vi "Build Type String.vi"(11 "App Build in":refnum<class "App Build.lvclass">) -> (2 "Build Type":string)   [LabVIEW 2020, in "Builder Tools.lvlib" / "App Build.lvclass"]
uses:
  App Build.lvclass
  App Build.lvclass/App Build.ctl
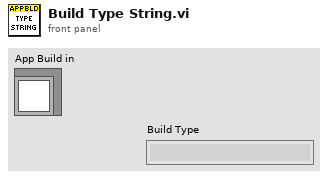
[diagram p1: front panel]
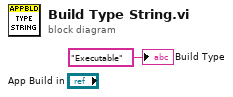
[diagram p0: block diagram]
diagram:
  "Build Type" <- "Executable" ("Build Type")
